vi "create socket.vi"(8 "error in":errorcluster, 10 "protocol":T1=80 items=["NN_PUSH"=80, "NN_PULL"=81, "NN_BUS"=112, "NN_PAIR"=16, "NN_PUB"=32, "NN_SUB"=33, "NN_REQ"=48, "NN_REP"=49, "NN_SURVEYOR"=96, "NN_RESPONDENT"=97], 11 "domain":T2=enum."AF_SP") -> (0 "error out":errorcluster, 3 "socket":i64)   [LabVIEW 2013, in "lvnano.lvlib"]
doc: "NN_EXPORT int nn_socket (int domain, int protocol);"
uses:
  lvnano.lvlib
  lvnanomsg.dll
  domain.ctl
  protocol.ctl
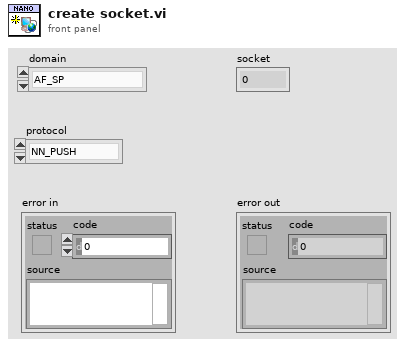
[diagram p1: front panel]
types:
  T1 = typedef "lvnano.lvlib/protocol.ctl" = i32
  T2 = typedef "lvnano.lvlib/domain.ctl" = enum16{"Invalid", "AF_SP", "AF_SP_RAW"}
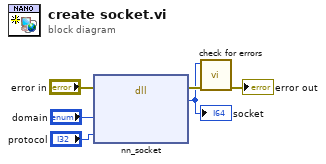
[diagram p0: block diagram]
diagram:
  n1 = dll-call lib="C:/Users/Daniel/Documents/nanomsg/lvnano/lvnanomsg.*" fn="nn_socket"(error in="error in", "domain"="domain", "protocol"="protocol") -> (error out=w3:errorcluster, "socket"=w1:i64)  [unwired: 4 in, 1 out]
  "socket" <- w1
  n2 = call "check for errors.vi"("error in"=w3, "function return"=w1) -> ("error out"=→"error out":errorcluster)  [unwired: 9 in]
